vi "NMEA_type.vi"(1 "NMEA String":string) -> (0 "NMEA Sentence Type":string)   [LabVIEW 2010]
uses:
  <vilib>/regexp/Match Regular Expression.xnode
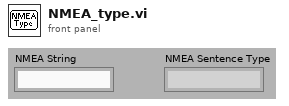
[diagram p1: front panel]
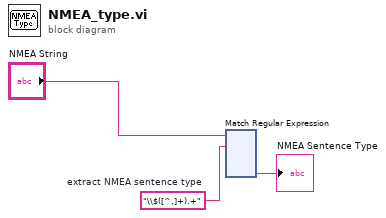
[diagram p0: block diagram]
diagram:
  w1 = "\\$([^,]+).+"  # extract NMEA sentence type
  n1 = xnode "Match Regular Expression"("input string"="NMEA String", "regular expression"=w1) -> ("submatch 1"=→"NMEA Sentence Type":string)  [unwired: 3 in, 6 out]
